vi "Error - Log File.vi"(8 "error in (no error)":errorcluster, 9 "Error Data":variant, 10 "Error Type":T1) -> (0 "error out":errorcluster)   [LabVIEW 2017]
doc: "This SubVI serves for maintain a log file with unknown errors.\n[Covers: EH2]"
uses:
  Controls/Error Type.ctl
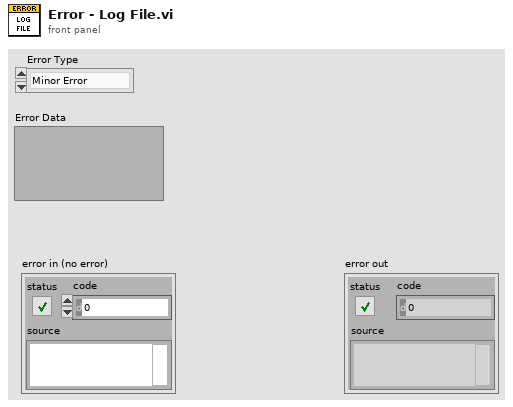
[diagram p1: front panel]
types:
  T1 = typedef "Error Type.ctl" = enum16{"Minor Error", "Wash Cycle Error", "System Error", "Unknown"}
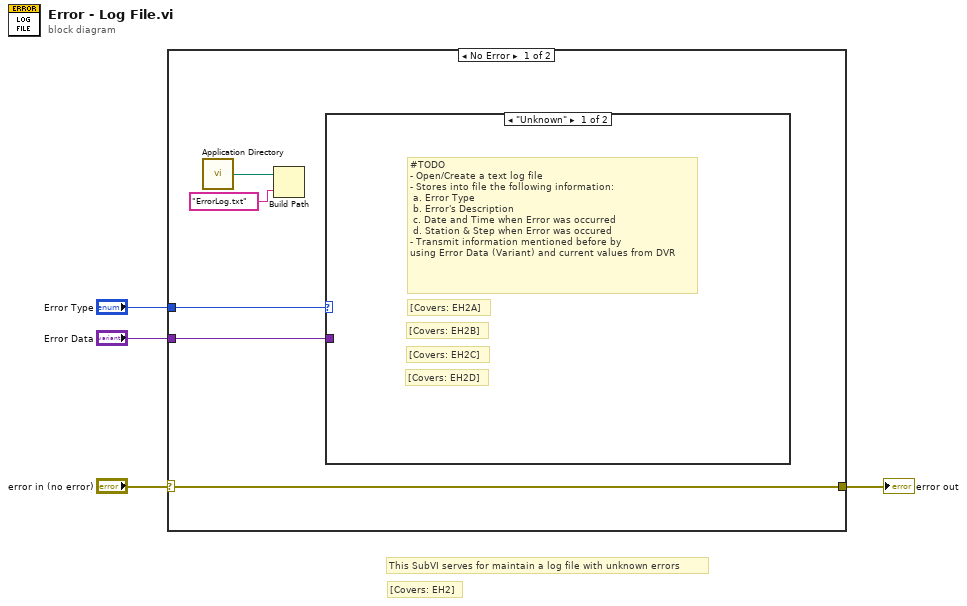
[diagram p0: block diagram]
diagram:
  # "[Covers: EH2]"
  # "This SubVI serves for maintain a log file with unknown errors"
  n1 = case shown="No Error" "error in (no error)" {
    selector: "error in (no error)" -> [w9 w10]
    tunnel: [w9 w10] -> w3
    tunnel: "Error Type" -> [w6 _]
    tunnel: "Error Data" -> [w5 _]
    frame No Error {
      n2 = call <vilib>:"Application Directory.vi"() -> ("Application Directory"=w8:path)
      n3 = Build Path(base path=w8, name or relative path="ErrorLog.txt") -> ()  [unwired: 1 out]
      n4 = case shown="\"Unknown\"" w6 {
        tunnel: w5 -> [_ _]
        frame "Unknown" {
          # "[Covers: EH2D]"
          # "[Covers: EH2C]"
          # "[Covers: EH2B]"
          # "[Covers: EH2A]"
          # "#TODO\n- Open/Create a text log file\n- Stores into file the following information:\n a. Error Type\n b. Error's Description\n c. Date and Time when Error was occurred\n d. Station & Step when Error was occured\n- Transmit information mentioned before by\nusing Error Data (Variant) and current values from DVR"
        }
        frame Default {
        }
      }
    }
    frame Error {
    }
  }
  "error out" <- w3
